vi "set_frequency.vi"(8 "error in":errorcluster, 11 "RF Generator settings":T2) -> (0 "error out":errorcluster)   [LabVIEW 2013, in "HP83712B_RF_Generator.lvclass"]
uses:
  HP83712B_RF_Generator.lvclass
  <vilib>/Instr/_visa.llb/GPIB Status Boolean Array.ctl
  RF_Generator_settings.ctl
  GPIB.lvclass
panel:
  out "FREQ string":string
  out "FREQ status":T1
  out "POW status":T1
  out "GPIB channel #":string
  out "POW string":string
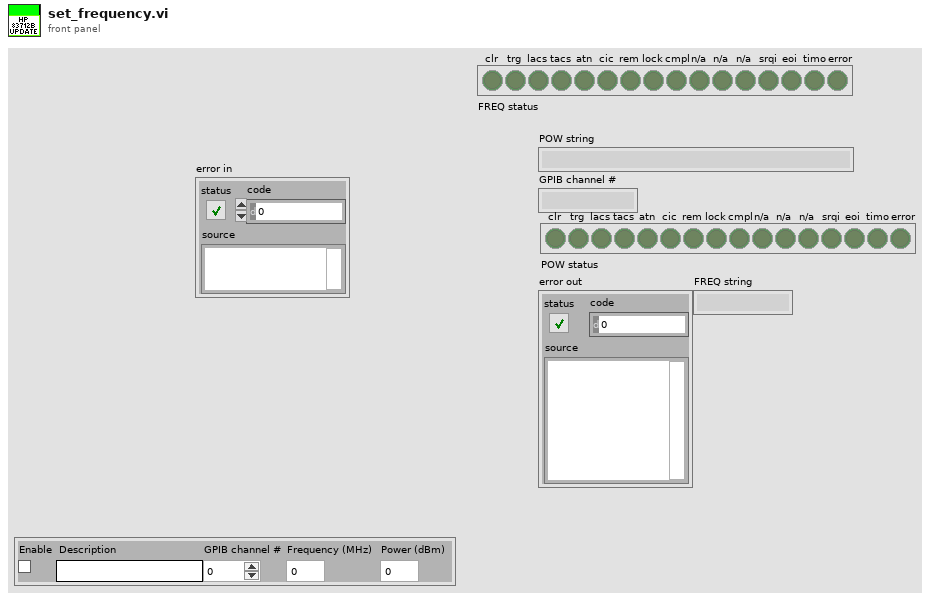
[diagram p1: front panel]
types:
  T1 = typedef "GPIB Status Boolean Array.ctl" = bool[]
  T2 = typedef "GPIB.lvclass/RF_Generator_settings.ctl" = cluster{"Enable":bool, "Description":string, "GPIB channel #":u8, "Frequency (MHz)":dbl, "Power (dBm)":dbl}
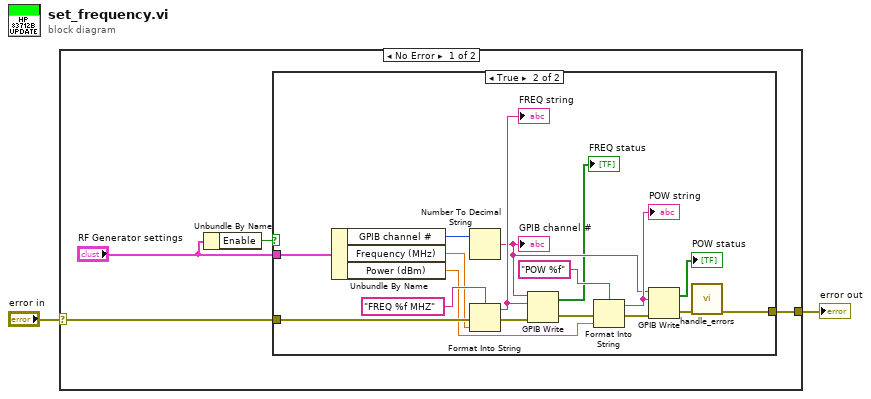
[diagram p0: block diagram]
diagram:
  n1 = case shown="No Error" "error in" {
    selector: "error in" -> [w4 w25]
    tunnel: [w3 w25] -> w1
    frame No Error {
      n2 = Unbundle By Name("RF Generator settings") -> ("Enable"=w5:bool)
      n3 = case shown="True" w5 {
        tunnel: "RF Generator settings" -> [_ w18]
        tunnel: w4 -> [w7 w11]
        tunnel: [w7 w17] -> w3
        frame False {
        }
        frame True {
          n4 = Unbundle By Name(w18) -> ("GPIB channel #"=w19:u8, "Frequency (MHz)"=w8:dbl, "Power (dBm)"=w9:dbl)
          n5 = Number To Decimal String(number=w19) -> (decimal integer string=w13:string)  [unwired: 1 in]
          "GPIB channel #" <- w13
          n6 = Format Into String(format string="FREQ %f MHZ", error in=w11, w8) -> (resulting string=w14:string, error out=w15:errorcluster)  [unwired: 1 in]
          "FREQ string" <- w14
          n7 = GPIB Write(0:w13, 1:w14, 3:w15) -> (5:→"FREQ status":bool[], 6:w10:errorcluster)  [unwired: 2 in]
          n8 = Format Into String(format string="POW %f", error in=w10, w9) -> (resulting string=w23:string, error out=w21:errorcluster)  [unwired: 1 in]
          "POW string" <- w23
          n9 = GPIB Write(0:w13, 1:w23, 3:w21) -> (5:→"POW status":bool[], 6:w20:errorcluster)  [unwired: 2 in]
          n10 = call "handle_errors.vi"("error in (no error)"=w20) -> ("error out"=w17:errorcluster)  [unwired: 14 in]
        }
      }
    }
    frame Error {
    }
  }
  "error out" <- w1
